vi "conv_Pos_Fre.vi"(6 "data_in":dbl[][](array[numeric]), 8 "error in":errorcluster, 11 "Pos":dbl=30.0) -> (0 "error out":errorcluster, 3 "FreQ":dbl, 4 "data_out":dbl[][](array[numeric]))   [LabVIEW 2019]
uses:
  <vilib>/Utility/file.llb/Read Delimited Spreadsheet (DBL).vi
  <vilib>/gmath/NI_Gmath.lvlib
panel:
  out "array_Freq":dbl[](array[numeric])
  out "array_Pos":dbl[](array[numeric])
  out "yi":dbl[](array[numeric]) format="%_6g"
  out "xi used":dbl[](array[numeric]) format="%_6g"
  # "VI to convert vapor pressure of He4 or He3 to temperature.\n\ndata_out can/should be fed back to data_in \nso as to read the data file only once."
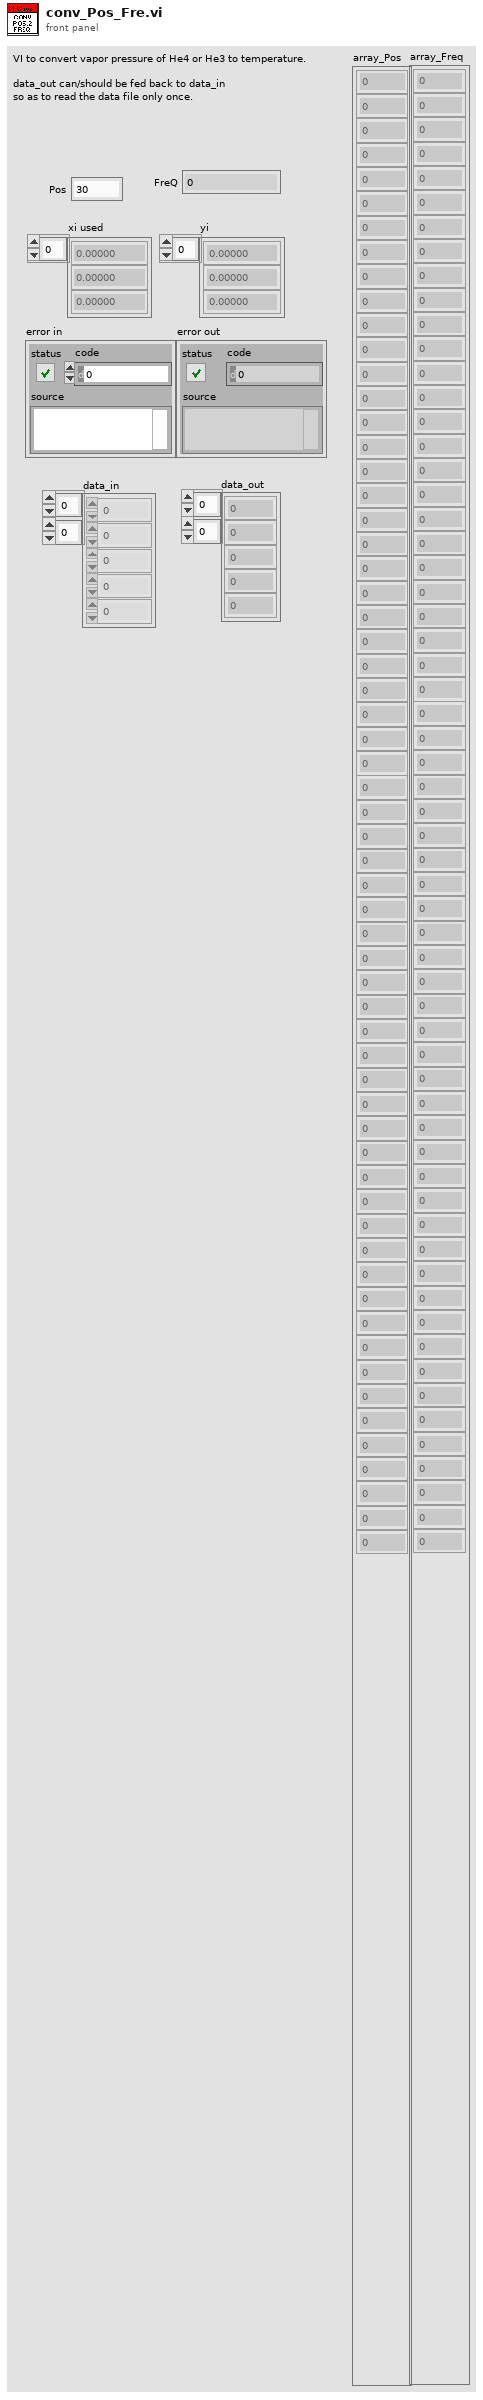
[diagram p1: front panel]
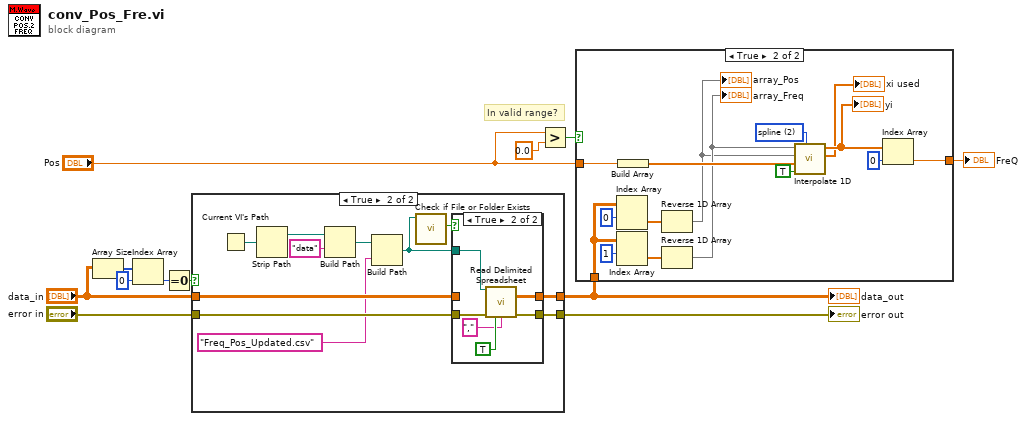
[diagram p0: block diagram]
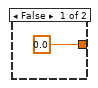
[diagram p2: hidden frame]
diagram:
  # "In valid range?"
  n1 = Array Size(array="data_in") -> (size(s)=w6:i32[])
  n2 = Index Array(array=w6, index=0) -> (element=w5:i32)
  n3 = Equal To 0?(x=w5) -> (x = 0?=w9:bool)
  n4 = case shown="True" w9 {
    tunnel: "error in" -> [w13 w19]
    tunnel: [w13 w18] -> w11
    tunnel: [w14 w17] -> w8
    tunnel: "data_in" -> [w14 w16]
    frame False {
    }
    frame True {
      n5 = Current VI's Path() -> (path=w25:path)
      n6 = Strip Path(path=w25) -> (stripped path=w24:path)  [unwired: 1 out]
      n7 = Build Path(base path=w24, name or relative path="data") -> (appended path=w22:path)
      n8 = Build Path(base path=w22, name or relative path="Freq_Pos_Updated.csv") -> (appended path=w20:path)
      n9 = call <vilib>:"Check if File or Folder Exists.vi"("path"=w20) -> ("file or folder exists?"=w21:bool)  [unwired: 8 in, 2 out]
      n10 = case shown="True" w21 {
        tunnel: w20 -> [_ w33]
        tunnel: w19 -> [w26 w32]
        tunnel: [w26 w31] -> w18
        tunnel: [w27 w30] -> w17
        tunnel: w16 -> [w27 _]
        frame False {
        }
        frame True {
          n11 = call-poly <vilib>:"Read Delimited Spreadsheet.vi"("file path (dialog if empty)"=w33, "error in (no error)"=w32, "transpose? (F)"=TRUE, "delimiter (\\t)"="," ("delimiter (\\t)")) -> ("all rows"=w30:dbl[][], "error out"=w31:errorcluster)  [unwired: 6 in, 4 out]
        }
      }
    }
  }
  "error out" <- w11
  "data_out" <- w8
  n12 = Greater?(x="Pos", y=0.0) -> (0:w1:bool)
  n13 = case shown="True" w1 {
    tunnel: w8 -> [_ w48]
    tunnel: [0.0 ("Numeric") w44] -> w7
    tunnel: "Pos" -> [_ w37]
    frame False {
    }
    frame True {
      w38 = 2 items=["nearest", "linear", "spline", "cubic Hermite", "Lagrange"] ("method")
      n14 = Index Array(array=w48, index (row)=0) -> (element=w41:dbl[])  [unwired: 1 in]
      n15 = Index Array(array=w48, index (row)=1) -> (element=w40:dbl[])  [unwired: 1 in]
      n16 = Build Array(w37) -> (w43:dbl[])
      n17 = Reverse 1D Array(array=w41) -> (reversed array=w35:dbl[])
      "array_Pos" <- w35
      n18 = Reverse 1D Array(array=w40) -> (reversed array=w36:dbl[])
      "array_Freq" <- w36
      n19 = call <vilib>:"Interpolate 1D.vi"("method"=w38, "X is monotonic"=TRUE, "xi"=w43, "X"=w35, "Y"=w36) -> ("xi used"=→"xi used":dbl[], "yi"=w46:dbl[])  [unwired: 4 in, 1 out]
      "yi" <- w46
      n20 = Index Array(array=w46, index=0) -> (element=w44:dbl)
    }
  }
  "FreQ" <- w7
